vi "Number of test runners.vi"() -> ()   [LabVIEW 2020]
uses:
  <vilib>/Astemes/LUnit/LUnit Method Result.lvclass/LUnit Method Result.ctl
  <vilib>/Astemes/LUnit/LUnit Method Result.lvclass
  <vilib>/Astemes/LUnit/LUnit Execution API.lvclass
panel:
  in  "Numbers of Test Runners":i32[](array[numeric])=[1, 2, 4, 8, 12, 16, 20, 24]
  out "Test Method Name":string
  out "Method count":u32
  out "Current number of test runners":i32
  out "Test Time as Function of Number of Test Runners":cluster{"Numeric":i32, dbl}[](graph)
  out "Tests Completed":bool
  out "Test times":dbl[](array[numeric])
  # "This VI runs all tests in its owning project and measures the execution times for each number of test runners. The execution times are expected to be faster than using the LUnit User Interface as there is less overhead using the API."
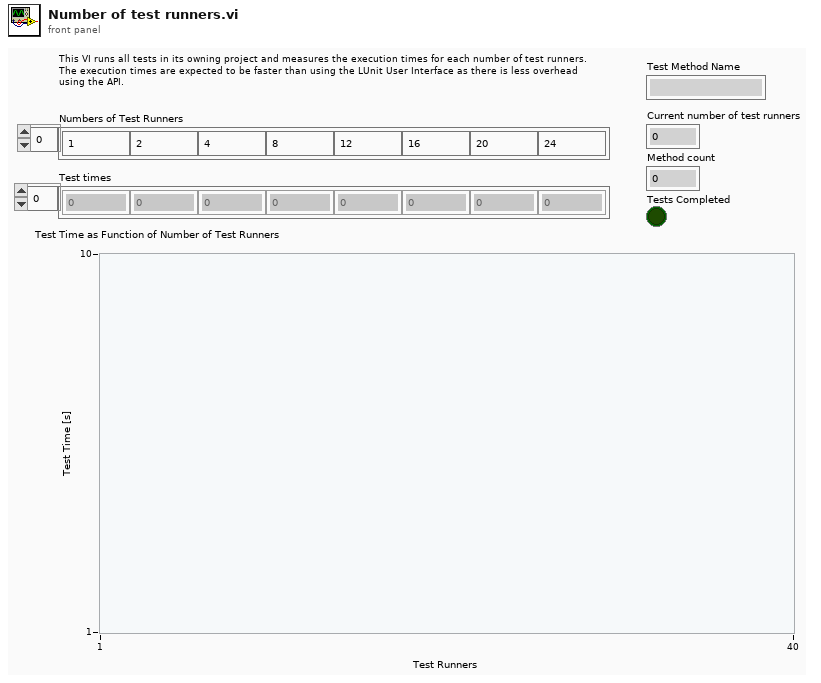
[diagram p1: front panel]
types:
  T1 = cluster{"Event Registration Refnum":refnum<event-registration>, "Event Registration Refnum":refnum<event-registration>}
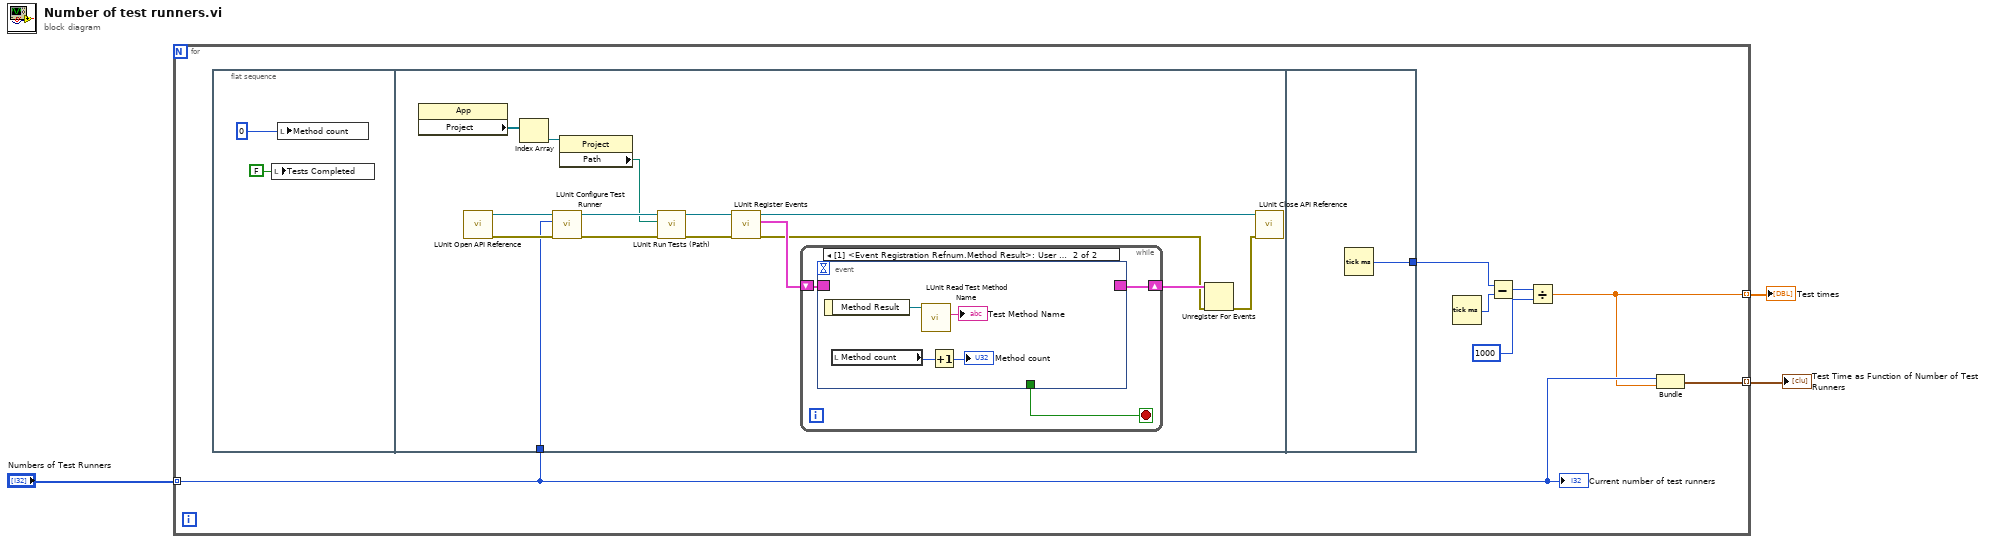
[diagram p0: block diagram]
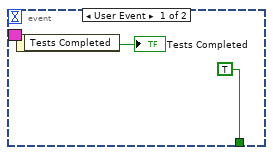
[diagram p2: hidden frame]
diagram:
  n1 = for {
    tunnel: [w5] -> w3 mode=indexing
    tunnel: "Numbers of Test Runners" -> [w6] mode=indexing
    tunnel: [w4] -> w2 mode=indexing
    n2 = flat-sequence {
      tunnel: w6 -> [w16]
      tunnel: [w37] -> w10
      frame #0 {
        n3 = local write "Tests Completed"(FALSE ("Tests Completed")) -> ()
        n4 = local write "Method count"(u32 0 ("Numeric")) -> ()
      }
      frame #1 {
        n5 = property class="App"() -> ("Project"=w15:refnum<vi>[])  [unwired: 2 in, 2 out]
        n6 = call <vilib>:"LUnit Open API Reference.vi"() -> ("error out"=w26:errorcluster, "Execution API out"=w27:refnum<class "LUnit Execution API.lvclass">)  [unwired: 10 in]
        n7 = Index Array(array=w15) -> (element=w14:refnum<vi>)  [unwired: 1 in]
        n8 = call <vilib>:"LUnit Configure Test Runner.vi"("error in (no error)"=w26, "Number of Test Runners"=w16, "Execution API In"=w27) -> ("error out"=w24:errorcluster, "Execution API Out"=w25:refnum<class "LUnit Execution API.lvclass">)  [unwired: 7 in]
        n9 = property class="Project"(reference=w14) -> ("Path"=w13:path)  [unwired: 1 in, 2 out]
        n10 = call <vilib>:"LUnit Run Tests (Path).vi"("error in (no error)"=w24, "Project or Class Path"=w13, "Execution API In"=w25) -> ("error out"=w22:errorcluster, "Execution API Out"=w23:refnum<class "LUnit Execution API.lvclass">)  [unwired: 7 in]
        n11 = call <vilib>:"LUnit Register Events.vi"("error in (no error)"=w22, "Execution API In"=w23) -> ("error out"=w18:errorcluster, "Result Events"=w21:T1, "Execution API Out"=w20:refnum<class "LUnit Execution API.lvclass">)  [unwired: 7 in]
        n12 = while {
          shift-right: [w29] -> w19
          shift-left: w21 -> [w30]
          stop <- w28 stop-if-true
          n13 = event shown="[1] <Event Registration Refnum.Method Result>: User Event" {
            selector: w30 -> [_ _]
            dyn-events: [_ _] -> w29
            timeout: _ -> [_ _]
            tunnel: [TRUE _] -> w28
            event User Event {
              n14 = event-data() -> ("Tests Completed"=→"Tests Completed":bool)  [unwired: 1 in]
            }
            event User Event {
              n15 = event-data() -> ("Method Result"=w33:refnum<class "LUnit Method Result.lvclass">)  [unwired: 1 in]
              n16 = local read "Method count"() -> (w34:u32)
              n17 = call <vilib>:"LUnit Read Test Method Name.vi"("Method Result In"=w33) -> ("Test Method Name"=→"Test Method Name":string)  [unwired: 9 in, 1 out]
              n18 = Increment(x=w34) -> (x+1=→"Method count":u32)
            }
          }
        }
        n19 = Unregister For Events(event registration refnum=w19, error in=w18) -> (error out=w17:errorcluster)
        n20 = call <vilib>:"LUnit Close API Reference.vi"("error in (no error)"=w17, "Execution API in"=w20) -> ()  [unwired: 9 in, 1 out]
      }
      frame #2 {
        n21 = Tick Count (ms)() -> (millisecond timer value=w37:u32)
      }
    }
    n22 = Tick Count (ms)() -> (millisecond timer value=w9:u32)
    n23 = Subtract(x=w10, y=w9) -> (x-y=w8:u32)
    n24 = Divide(x=w8, y=u32 1000) -> (x/y=w5:dbl)
    n25 = Bundle("Numeric"=w6, w5) -> (w4:cluster{"Numeric":i32, dbl})  [unwired: 1 in]
    "Current number of test runners" <- w6
  }
  "Test times" <- w3
  "Test Time as Function of Number of Test Runners" <- w2
